vi "Polish BD Constant.vi"(10 "BD Const":refnum<vi>, 11 "Array Writer in":refnum<class "Array Writer.lvclass">) -> (3 "Array Writer out":refnum<class "Array Writer.lvclass">)   [LabVIEW 2013, in "Array Writer.lvclass"]
doc: "Copyright (c) 2016 Sze Howe Koh\n\nThis Source Code Form is subject to the terms of the Mozilla Public License, v. 2.0. If a copy of the MPL was not distributed with this file, You can obtain one at http://mozilla.org/MPL/2.0/."
uses:
  Array Writer.lvclass
  Array Writer.lvclass/Array Writer.ctl
  Abstract Param Writer/Abstract Param Writer.lvclass
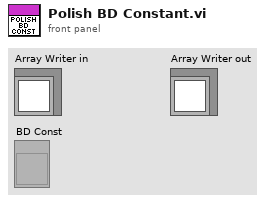
[diagram p1: front panel]
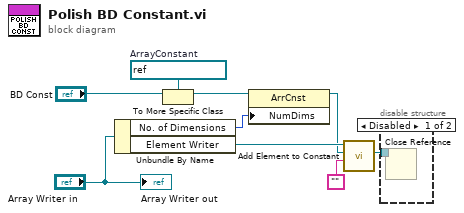
[diagram p0: block diagram]
diagram:
  w6 = refnum<vi> refnum  # ArrayConstant
  n1 = Unbundle By Name("Array Writer in") -> ("No. of Dimensions"=w2:u32, "Element Writer"=w9:refnum<class "Abstract Param Writer.lvclass">)
  n2 = To More Specific Class(target class=w6, reference="BD Const") -> (specific class reference=w4:refnum<vi>)  [unwired: 1 in, 1 out]
  n3 = property class="ArrCnst"(reference=w4, "NumDims"=w2) -> (reference out=w3:refnum<vi>)  [unwired: 1 in, 1 out]
  n4 = call-dynamic "Add Element to Constant.vi"("Element Name"="", "Cluster or Array"=w3, "Abstract Param Writer in"=w9) -> ("Cluster or Array Dup"=w1:refnum<vi>)  [unwired: 7 in, 1 out]
  n5 = disable-structure shown="Disabled" {
    disable-tunnel: w1 -> [w10 _]
    frame Disabled {
      n6 = Close Reference(reference=w10) -> ()  [unwired: 1 in, 1 out]
    }
    frame Enabled {
    }
  }
  "Array Writer out" <- "Array Writer in"
